vi "Auto_Routine_Cube_Backup_Cone.vi"(8 "error in (no error)":errorcluster) -> (0 "error out":errorcluster)   [LabVIEW 2020]
uses:
  Arm/ArmPositionPreset.ctl
  <vilib>/Rock Robotics/WPI/DriverStation/WPI_DriverStationAllianceInfo.ctl
  Arm/ArmGamePiecePreset.ctl
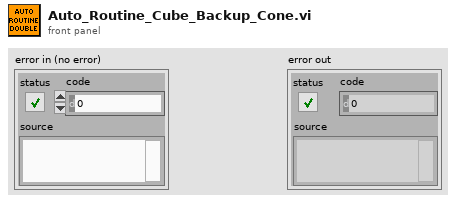
[diagram p1: front panel]
types:
  T1 = typedef "ArmGamePiecePreset.ctl" = enum16{"Cube", "Cone"}
  T2 = typedef "ArmPositionPreset.ctl" = enum16{"Upper", "Lower", "Middle", "Home", "Shelf", "Floor", "HalfFloor", "HalfHome"}
  T3 = typedef "WPI_DriverStationAllianceInfo.ctl" = enum16{"Red", "Blue", "Invalid"}
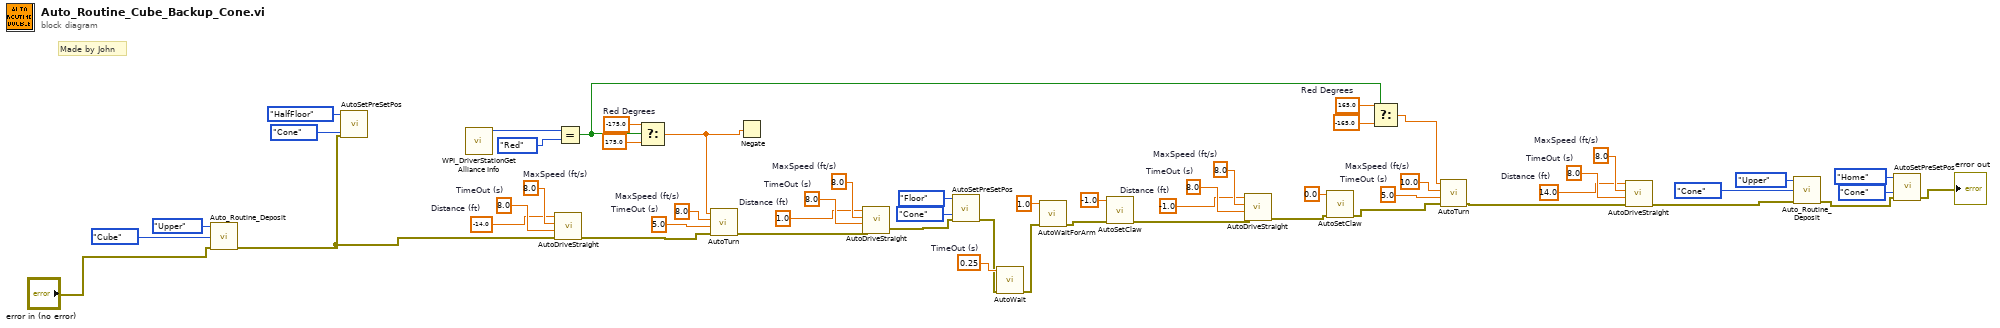
[diagram p0: block diagram]
diagram:
  w3 = 0.25  # TimeOut (s)
  w13 = 165.0  # Red Degrees
  w19 = 8.0  # TimeOut (s)
  w20 = 8.0  # MaxSpeed (ft/s)
  w18 = 14.0  # Distance (ft)
  w22 = 5.0  # TimeOut (s)
  w23 = 10.0  # MaxSpeed (ft/s)
  w28 = 8.0  # TimeOut (s)
  w29 = 8.0  # MaxSpeed (ft/s)
  w27 = -1.0  # Distance (ft)
  w34 = 8.0  # TimeOut (s)
  w35 = 8.0  # MaxSpeed (ft/s)
  w33 = 1.0  # Distance (ft)
  w36 = -175.0  # Red Degrees
  w41 = 5.0  # TimeOut (s)
  w42 = 8.0  # MaxSpeed (ft/s)
  w53 = 8.0  # TimeOut (s)
  w54 = 8.0  # MaxSpeed (ft/s)
  w52 = -14.0  # Distance (ft)
  # "Made by John"
  n1 = call "Auto_Routine_Deposit.vi"("error in (no error)"="error in (no error)", "Game Piece"=ArmGamePiecePreset."Cube", "Position"=ArmPositionPreset."Upper") -> ("error out"=w5:errorcluster)  [unwired: 8 in]
  n2 = call "AutoSetPreSetPos.vi"("error in (no error)"=w5, "Game Piece"=ArmGamePiecePreset."Cone", "Position"=ArmPositionPreset."HalfFloor") -> ()  [unwired: 8 in, 1 out]
  n3 = call <vilib>:"WPI_DriverStationGet Alliance Info.vi"() -> ("Alliance"=w39:T3)  [unwired: 6 in, 5 out]
  n4 = call "AutoDriveStraight.vi"("error in (no error)"=w5, "TimeOut (s)"=w53, "MaxSpeed (ft/s)"=w54, "Dist (ft)"=w52) -> ("error out"=w40:errorcluster)  [unwired: 7 in]
  n5 = Equal?(x=w39, y=WPI_DriverStationAllianceInfo."Red") -> (x = y?=w11:bool)
  n6 = Select(t=w36, s=w11, f=175.0) -> (s? t:f=w24:dbl)
  n7 = call "AutoTurn.vi"("error in (no error)"=w40, "TimeOut (s)"=w41, "MaxSpeed (ft/s)"=w42, "degrees"=w24) -> ("error out"=w32:errorcluster)  [unwired: 7 in]
  n8 = Negate(x=w24) -> ()  [unwired: 1 out]
  n9 = call "AutoDriveStraight.vi"("error in (no error)"=w32, "TimeOut (s)"=w34, "MaxSpeed (ft/s)"=w35, "Dist (ft)"=w33) -> ("error out"=w31:errorcluster)  [unwired: 7 in]
  n10 = call "AutoSetPreSetPos.vi"("error in (no error)"=w31, "Game Piece"=ArmGamePiecePreset."Cone", "Position"=ArmPositionPreset."Floor") -> ("error out"=w2:errorcluster)  [unwired: 8 in]
  n11 = call "AutoWait.vi"("error in (no error)"=w2, "TimeOut (s)"=w3) -> ("error out"=w1:errorcluster)  [unwired: 9 in]
  n12 = call "AutoWaitForArm.vi"("error in (no error)"=w1, "TimeOut (s)"=1.0) -> ("error out"=w30:errorcluster)  [unwired: 9 in]
  n13 = call "AutoSetClaw.vi"("error in (no error)"=w30, "ClawDemand"=-1.0) -> ("error out"=w26:errorcluster)  [unwired: 9 in]
  n14 = call "AutoDriveStraight.vi"("error in (no error)"=w26, "TimeOut (s)"=w28, "MaxSpeed (ft/s)"=w29, "Dist (ft)"=w27) -> ("error out"=w25:errorcluster)  [unwired: 7 in]
  n15 = call "AutoSetClaw.vi"("error in (no error)"=w25, "ClawDemand"=0.0) -> ("error out"=w21:errorcluster)  [unwired: 9 in]
  n16 = Select(t=w13, s=w11, f=-165.0) -> (s? t:f=w12:dbl)
  n17 = call "AutoTurn.vi"("error in (no error)"=w21, "TimeOut (s)"=w22, "MaxSpeed (ft/s)"=w23, "degrees"=w12) -> ("error out"=w17:errorcluster)  [unwired: 7 in]
  n18 = call "AutoDriveStraight.vi"("error in (no error)"=w17, "TimeOut (s)"=w19, "MaxSpeed (ft/s)"=w20, "Dist (ft)"=w18) -> ("error out"=w10:errorcluster)  [unwired: 7 in]
  n19 = call "Auto_Routine_Deposit.vi"("error in (no error)"=w10, "Game Piece"=ArmGamePiecePreset."Cone", "Position"=ArmPositionPreset."Upper") -> ("error out"=w7:errorcluster)  [unwired: 8 in]
  n20 = call "AutoSetPreSetPos.vi"("error in (no error)"=w7, "Game Piece"=ArmGamePiecePreset."Cone", "Position"=ArmPositionPreset."Home") -> ("error out"=→"error out":errorcluster)  [unwired: 8 in]
